vi "Load VI.vi"(4 "Control[] (Empty: all)":refnum<vi>[](array[refnum]), 6 "Section Name (\"Settings\")":string="Settings", 7 "Restore in Dev Environment? (F)":bool, 8 "error in (no error)":errorcluster, 9 "Path (Prefix:Top Level Name.ini)":path, 10 "VI Reference In (Caller)":refnum<vi>, 11 "Save Restore Settings in":refnum<class "Save Restore Settings.lvclass">) -> (0 "error out":errorcluster, 2 "VI Reference Out":refnum<vi>, 3 "Save Restore Settings out":refnum<class "Save Restore Settings.lvclass">)   [LabVIEW 2020, in "Save Restore Settings.lvclass"]
doc: "Loads the settings associated with a VI, including panel bounds, splitter bar positions, listbox column widths, and graph/chart plots. The settings are saved in an ini file at the specified path. The <B>Save Restore Settings in</B> class may be supplied with a child class to customize what properties are saved. Other notes:\nThis VI does not load settings by default if the development environment is used. This is so changes made at edit time will not be overwritten by the last saved settings when a VI is run.\nAutoscale, legend visibility, and other graph/chart settings that affect usability are not saved by default. \nIf executable windows with unlocked splitters are built with a larger front panels than the panel sizes specified by the settings file, redraw issues may occur. To avoid this, build executables with windows at their minimum size.\n\nAuthored by Shawn Walpole\nsupport@mooregoodideas.com\nwww.mooregoodideas.com\n\nCopyright (c) 2010, Moore Good Ideas, Inc.\n\nAll rights reserved.\n\nRedistribution and use in source and binary forms, with or without modification, are permitted provided that the following conditions are met:\n\n * Redistributions of source code must retain the above copyright notice, this list of conditions and the following disclaimer.\n * Redistributions in binary form must reproduce the above copyright notice, this list of conditions and the following disclaimer in the documentation and/or other materials provided with the distribution.\n * Neither the name of Moore Good Ideas, Inc. nor the names of its contributors may be used to endorse or promote products derived from this software without specific prior written permission.\n\nTHIS SOFTWARE IS PROVIDED BY THE COPYRIGHT HOLDERS AND CONTRIBUTORS \"AS IS\" AND ANY EXPRESS OR IMPLIED WARRANTIES, INCLUDING, BUT NOT LIMITED TO, THE IMPLIED WARRANTIES OF MERCHANTABILITY AND FITNESS FOR A PARTICULAR PURPOSE ARE DISCLAIMED. IN NO EVENT SHALL THE COPYRIGHT OWNER OR CONTRIBUTORS BE LIABLE FOR ANY DIRECT, INDIRECT, INCIDENTAL, SPECIAL, EXEMPLARY, OR CONSEQUENTIAL DAMAGES (INCLUDING, BUT NOT LIMITED TO, PROCUREMENT OF SUBSTITUTE GOODS OR SERVICES; LOSS OF USE, DATA, OR PROFITS; OR BUSINESS INTERRUPTION) HOWEVER CAUSED AND ON ANY THEORY OF LIABILITY, WHETHER IN CONTRACT, STRICT LIABILITY, OR TORT (INCLUDING NEGLIGENCE OR OTHERWISE) ARISING IN ANY WAY OUT OF THE USE OF THIS SOFTWARE, EVEN IF ADVISED OF THE POSSIBILITY OF SUCH DAMAGE."
uses:
  <userlib>/_MGI/Application Control/MGI Save Restore Settings/Save Restore Settings.lvclass
  <userlib>/_MGI/Application Control/MGI VI Reference/MGI Caller's VI Reference.vi
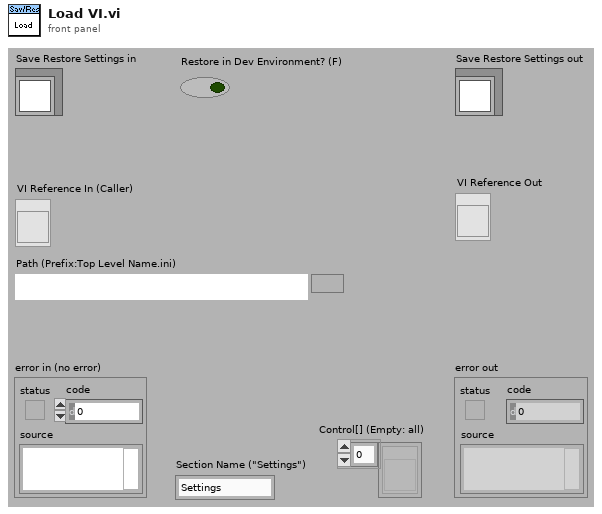
[diagram p1: front panel]
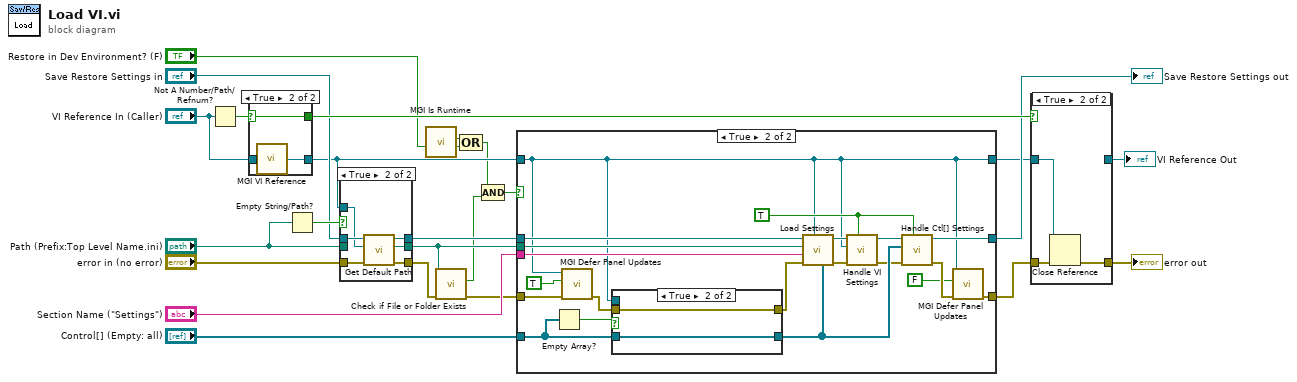
[diagram p0: block diagram]
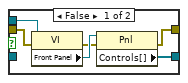
[diagram p3: hidden frame]
diagram:
  n1 = Not A Number/Path/Refnum?(number/path/refnum="VI Reference In (Caller)") -> (NaN/Path/Refnum?=w20:bool)
  n2 = case shown="True" w20 {
    selector: w20 -> [_ w26]
    tunnel: [w25 w27] -> w11
    tunnel: "VI Reference In (Caller)" -> [w25 _]
    tunnel: [_ w26] -> w23
    frame False {
    }
    frame True {
      n3 = call-poly <userlib>:"MGI VI Reference.vi"() -> ("Caller's VI Reference"=w27:refnum<vi>)  [unwired: 1 in]
    }
  }
  n4 = Empty String/Path?(string/path="Path (Prefix:Top Level Name.ini)") -> (empty?=w15:bool)
  n5 = case shown="True" w15 {
    tunnel: "error in (no error)" -> [w28 w36]
    tunnel: [w28 w35] -> w10
    tunnel: "Path (Prefix:Top Level Name.ini)" -> [w30 _]
    tunnel: "Save Restore Settings in" -> [w29 w34]
    tunnel: [w29 w33] -> w12
    tunnel: [w30 w32] -> w9
    tunnel: w11 -> [_ w31]
    frame False {
    }
    frame True {
      n6 = call-dynamic "Get Default Path.vi"("error in (no error)"=w36, "VI Refnum"=w31, "Save Restore Settings in"=w34) -> ("error out"=w35:errorcluster, "Default Path"=w32:path, "Save Restore Settings out"=w33:refnum<class "Save Restore Settings.lvclass">)  [unwired: 6 in]
    }
  }
  n7 = call <userlib>:"MGI Is Runtime.vi"() -> ("Run Time System?"=w2:bool)  [unwired: 7 in]
  n8 = call <vilib>:"Check if File or Folder Exists.vi"("error in (no error)"=w10, "path"=w9) -> ("error out"=w8:errorcluster, "file or folder exists?"=w6:bool)  [unwired: 7 in, 1 out]
  n9 = Compound Arithmetic op=OR(w2, "Restore in Dev Environment? (F)") -> (w3:bool)
  n10 = Compound Arithmetic op=AND(w3, w6) -> (w5:bool)
  n11 = case shown="True" w5 {
    tunnel: "Section Name (\"Settings\")" -> [_ w59]
    tunnel: [w37 w51] -> w18
    tunnel: [w38 w56] -> w17
    tunnel: w12 -> [w38 w54]
    tunnel: w11 -> [w39 w40]
    tunnel: w9 -> [_ w53]
    tunnel: w8 -> [w37 w49]
    tunnel: [w39 w40] -> w7
    tunnel: "Control[] (Empty: all)" -> [_ w46]
    frame False {
    }
    frame True {
      w55 = TRUE ("Write? (F:Read)")
      n12 = Empty Array?(array=w46) -> (empty?=w47:bool)
      n13 = call <userlib>:"MGI Defer Panel Updates.vi"("Error In"=w49, "Defer Updates?"=TRUE, "VI Reference (Caller)"=w40) -> ("Error Out"=w44:errorcluster)  [unwired: 8 in]
      n14 = case shown="True" w47 {
        tunnel: w44 -> [w63 w66]
        tunnel: [w62 w66] -> w43
        tunnel: [w61 w67] -> w42
        tunnel: w40 -> [w60 _]
        tunnel: w46 -> [_ w67]
        frame False {
          n15 = property class="VI"(reference=w60, error in=w63) -> (error out=w64:errorcluster, "Front Panel"=w65:refnum<vi>)  [unwired: 1 out]
          n16 = property class="Pnl"(reference=w65, error in=w64) -> (error out=w62:errorcluster, "Controls[]"=w61:refnum<vi>[])  [unwired: 1 out]
        }
        frame True {
        }
      }
      n17 = call-dynamic "Load Settings.vi"("Controls[]"=w42, "VI Refnum"=w40, "error in (no error)"=w43, "Section"=w59, "Path"=w53, "Save Restore Settings in"=w54) -> ("error out"=w45:errorcluster, "Save Restore Settings out"=w58:refnum<class "Save Restore Settings.lvclass">)  [unwired: 4 in]
      n18 = call-dynamic "Handle VI Settings.vi"("Write VI? (F:Read)"=w55, "error in (no error)"=w45, "VI Refnum"=w40, "Save Restore Settings in"=w58) -> ("error out"=w41:errorcluster, "Save Restore Settings out"=w57:refnum<class "Save Restore Settings.lvclass">)  [unwired: 6 in]
      n19 = call-dynamic "Handle Ctl[] Settings.vi"("Write Ctl? (F:Read)"=w55, "error in (no error)"=w41, "Controls[]"=w42, "Save Restore Settings in"=w57) -> ("error out"=w52:errorcluster, "Save Restore Settings out"=w56:refnum<class "Save Restore Settings.lvclass">)  [unwired: 6 in]
      n20 = call <userlib>:"MGI Defer Panel Updates.vi"("Error In"=w52, "Defer Updates?"=FALSE, "VI Reference (Caller)"=w40) -> ("Error Out"=w51:errorcluster)  [unwired: 8 in]
    }
  }
  "Save Restore Settings out" <- w17
  n21 = case shown="True" w23 {
    tunnel: w18 -> [w69 w72]
    tunnel: [w69 w70] -> w22
    tunnel: w7 -> [w68 w71]
    tunnel: [w68 _] -> w21
    frame False {
    }
    frame True {
      n22 = Close Reference(reference=w71, error in (no error)=w72) -> (error out=w70:errorcluster)
    }
  }
  "error out" <- w22
  "VI Reference Out" <- w21
